vi "Ic Distribution_DAQ_gate.vi"() -> ()   [LabVIEW 2017]
uses:
  global.vi
  <vilib>/Analysis/NI_AALBase.lvlib
panel:
  in  "Tab Control":enum32{"AWG", "DAQ", "Curve", "Error"}(tab)=enum."DAQ"
  in  "VISA resource name":refnum<visa-resource-name>="GPIB0::1::INSTR"
  in  "Sampling Frequency Hz":u64=10000000
  in  "End time S":dbl=0.005
  in  "Delay time S":dbl=0.3
  in  "Ramp time S":dbl=0.01
  in  "Amplitude V":dbl=5.0 format="%#_13g"
  in  "Channel Name":u16(ring)=1 items=["1"=1, "2"=2, "3"=3, "4"=4]
  in  "Update Wave":bool=TRUE
  in  "Points Number":i32=500
  in  "Gate":tag="Dev1/ao0"
  in  "Voltage Read":tag="Dev1/ai1"
  in  "Sample Rate":dbl=1000000.0 format="%.3p"
  in  "Trigger Level":dbl=0.1 format="%#_13g"
  in  "device in":tag="Dev1"
  out "Points get":i32=5000
  in  "intervals":i32=100
  out "Histogram Graph":T1(graph)={"X Values"=[1.3335459541621144, 1.3348573631903649, 1.3361687722186153, 1.3374801812468657, 1.3387915902751162, 1.3401029993033666, 1.341414408331617, 1.3427258173598675, 1.344037226388118, 1.3453486354163684, 1.3466600444446188, 1.3479714534728693, 1.3492828625011197, 1.3505942715293702, 1.3519056805576206, 1.353217089585871, 1.3545284986141215, 1.355839907642372, 1.3571513166706224, 1.3584627256988728, 1.3597741347271233, 1.3610855437553737, 1.3623969527836242, 1.3637083618118746, 1.365019770840125, 1.3663311798683755, 1.367642588896626, 1.3689539979248764, 1.3702654069531268, 1.3715768159813773, 1.3728882250096277, 1.3741996340378781, 1.3755110430661286, 1.376822452094379, 1.3781338611226295, 1.37944527015088, 1.3807566791791304, 1.3820680882073808, 1.3833794972356313, 1.3846909062638817, 1.3860023152921321, 1.3873137243203826, 1.388625133348633, 1.3899365423768835, 1.391247951405134, 1.3925593604333844, 1.3938707694616348, 1.3951821784898852, 1.3964935875181357, 1.3978049965463861, 1.3991164055746366, 1.400427814602887, 1.4017392236311375, 1.403050632659388, 1.4043620416876383, 1.4056734507158888, 1.4069848597441392, 1.4082962687723897, 1.4096076778006401, 1.4109190868288906, 1.412230495857141, 1.4135419048853914, 1.4148533139136419, 1.4161647229418923, 1.4174761319701428, 1.4187875409983932, 1.4200989500266437, 1.421410359054894, 1.4227217680831445, 1.424033177111395, 1.4253445861396454, 1.4266559951678959, 1.4279674041961463, 1.4292788132243968, 1.4305902222526472, 1.4319016312808976, 1.433213040309148, 1.4345244493373985, 1.435835858365649, 1.4371472673938994, 1.4384586764221499, 1.4397700854504003, 1.4410814944786507, 1.4423929035069012, 1.4437043125351516, 1.445015721563402, 1.4463271305916525, 1.447638539619903, 1.4489499486481534, 1.4502613576764039, 1.4515727667046543, 1.4528841757329047, 1.4541955847611552, 1.4555069937894056, 1.456818402817656, 1.4581298118459065, 1.459441220874157, 1.4607526299024074, 1.4620640389306578, 1.4633754479589083], "Histogram: h(x)"=[1, 0, 0, 0, 0, 0, 0, 0, 0, 0, 0, 0, 0, 0, 0, 0, 0, 0, 0, 0, 0, 0, 0, 0, 0, 0, 0, 0, 0, 0, 0, 0, 0, 0, 0, 0, 0, 0, 0, 0, 0, 0, 0, 0, 0, 0, 0, 0, 0, 0, 0, 0, 1, 2, 0, 0, 0, 0, 1, 2, 2, 2, 4, 4, 10, 12, 8, 14, 19, 15, 27, 41, 56, 77, 73, 95, 133, 147, 191, 208, 218, 275, 292, 337, 357, 423, 345, 321, 302, 262, 210, 181, 176, 61, 38, 29, 13, 5, 7, 3]}
  in  "stop":bool
  in  "error in no error":errorcluster
  out "error out":errorcluster
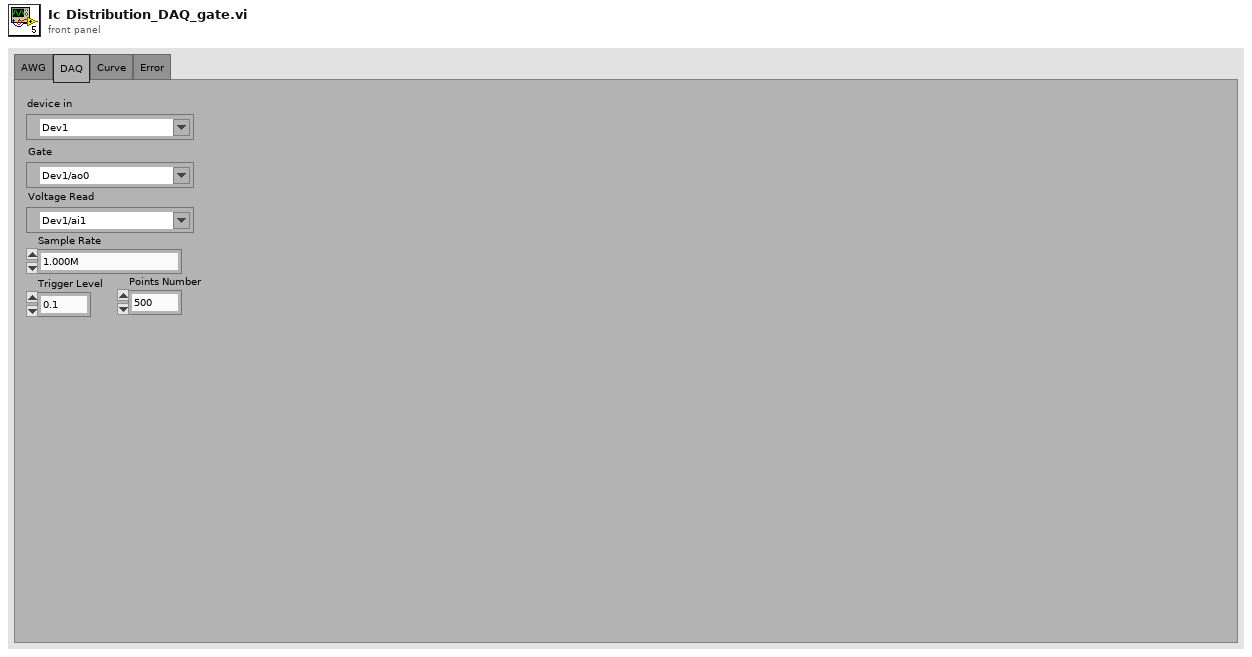
[diagram p1: front panel]
types:
  T1 = cluster{"X Values":dbl[], "Histogram: h(x)":i32[]}
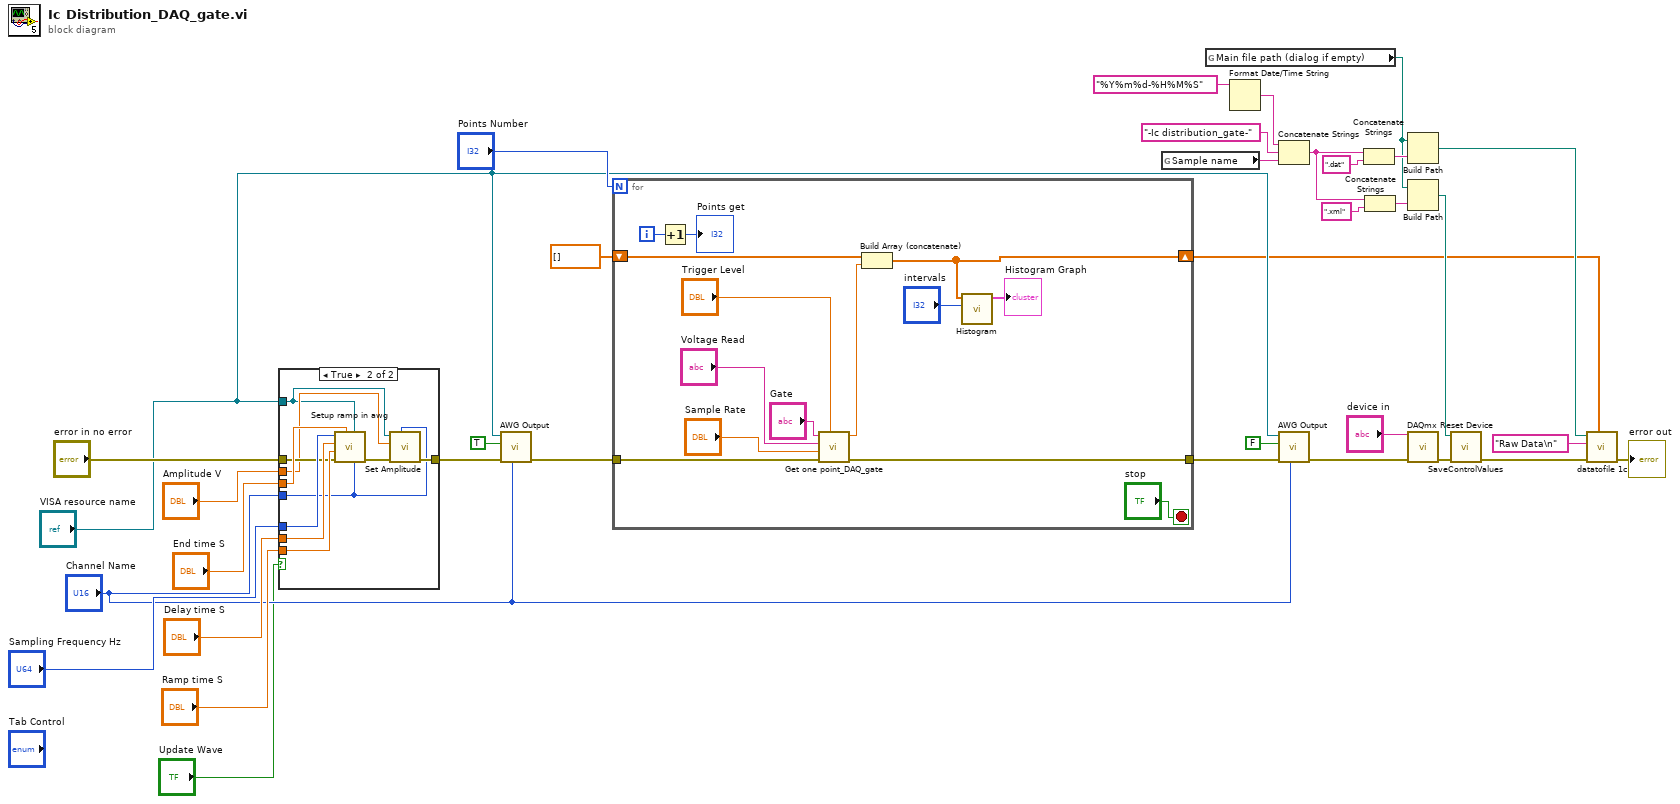
[diagram p0: block diagram]
diagram:
  n1 = case shown="True" "Update Wave" {
    tunnel: "Sampling Frequency Hz" -> [_ w46]
    tunnel: "End time S" -> [_ w45]
    tunnel: "Delay time S" -> [_ w44]
    tunnel: "Ramp time S" -> [_ w43]
    tunnel: "error in no error" -> [w36 w42]
    tunnel: "Amplitude V" -> [_ w41]
    tunnel: [w36 w39] -> w29
    tunnel: "Channel Name" -> [_ w38]
    tunnel: "VISA resource name" -> [_ w37]
    frame False {
    }
    frame True {
      n2 = call "Setup ramp in awg.vi"("Channel Name (1)"=w38, "VISA resource name"=w37, "End time S"=w45, "error in (no error)"=w42, "Ramp time S"=w43, "Delay time S"=w44, "Sampling Frequency (Hz)"=w46) -> ("error out"=w40:errorcluster)  [unwired: 4 in]
      n3 = call "Set Amplitude.vi"("Channel Name (1)"=w38, "error in (no error)"=w40, "Amplitude V"=w41, "VISA resource name"=w37) -> ("error out"=w39:errorcluster)  [unwired: 7 in]
    }
  }
  n4 = call "AWG Output.vi"("Channel Name (1)"="Channel Name", "error in (no error)"=w29, "Enable Output (T: Enable)"=TRUE, "VISA resource name"="VISA resource name") -> ("error out"=w26:errorcluster)  [unwired: 7 in]
  n5 = for {
    N: "Points Number" -> [_]
    tunnel: w26 -> [w58]
    shift-right: [w50] -> w2
    shift-left: dbl[] [] -> [w54]
    tunnel: [w53] -> w24
    i -> [w51]
    stop <- "stop" stop-if-true
    n6 = Increment(x=w51) -> (x+1=→"Points get":i32)
    n7 = call "Get one point_DAQ_gate.vi"("level"="Trigger Level", "error in (no error)"=w58, "Sample Rate"="Sample Rate", "Voltage Read"="Voltage Read", "Gate"="Gate") -> ("error out"=w53:errorcluster, "data"=w55:dbl)  [unwired: 5 in]
    n8 = Build Array (concatenate)(w54, w55) -> (w50:dbl[])
    n9 = call <vilib>:"Histogram.vi"("intervals"="intervals", "X"=w50) -> ("Histogram Graph"=→"Histogram Graph":T1)  [unwired: 6 in, 3 out]
  }
  n10 = global read "global.vi" "Sample name"() -> (w13:string)
  n11 = global read "global.vi" "Main file path (dialog if empty)"() -> (w8:path)
  n12 = Format Date/Time String(time format string (%c)="%Y%m%d-%H%M%S") -> (date/time string=w15:string)  [unwired: 2 in]
  n13 = Concatenate Strings(w15, "-Ic distribution_gate-" ("string"), w13) -> (w10:string)
  n14 = call "AWG Output.vi"("Channel Name (1)"="Channel Name", "error in (no error)"=w24, "Enable Output (T: Enable)"=FALSE, "VISA resource name"="VISA resource name") -> ("error out"=w20:errorcluster)  [unwired: 7 in]
  n15 = Concatenate Strings(w10, ".dat" ("string")) -> (w11:string)
  n16 = Concatenate Strings(w10, ".xml" ("string")) -> (w7:string)
  n17 = Build Path(base path=w8, name or relative path=w11) -> (appended path=w4:path)
  n18 = Build Path(base path=w8, name or relative path=w7) -> (appended path=w6:path)
  n19 = call <vilib>:"DAQmx Reset Device.vi"("device in"="device in", "error in"=w20) -> ("error out"=w3:errorcluster)  [unwired: 13 in]
  n20 = call "SaveControlValues.vi"("XML File Path"=w6, "error in (no error)"=w3) -> ("error out"=w5:errorcluster)  [unwired: 8 in]
  n21 = call "datatofile 1c.vi"("A1"=w2, "error in"=w5, "title"="Raw Data\n", "file path (dialog if empty)"=w4) -> ("error out"=→"error out":errorcluster)  [unwired: 7 in]
